vi "VERIFY DATA.vi"(11 "DATA IN":T1[](array[typedef])) -> (2 "DATA BAD?":bool, 3 "DATA OUT":T1[](array[typedef]))   [LabVIEW 2019]
uses:
  Controls/Table Data Types/Inventory Data Type.ctl
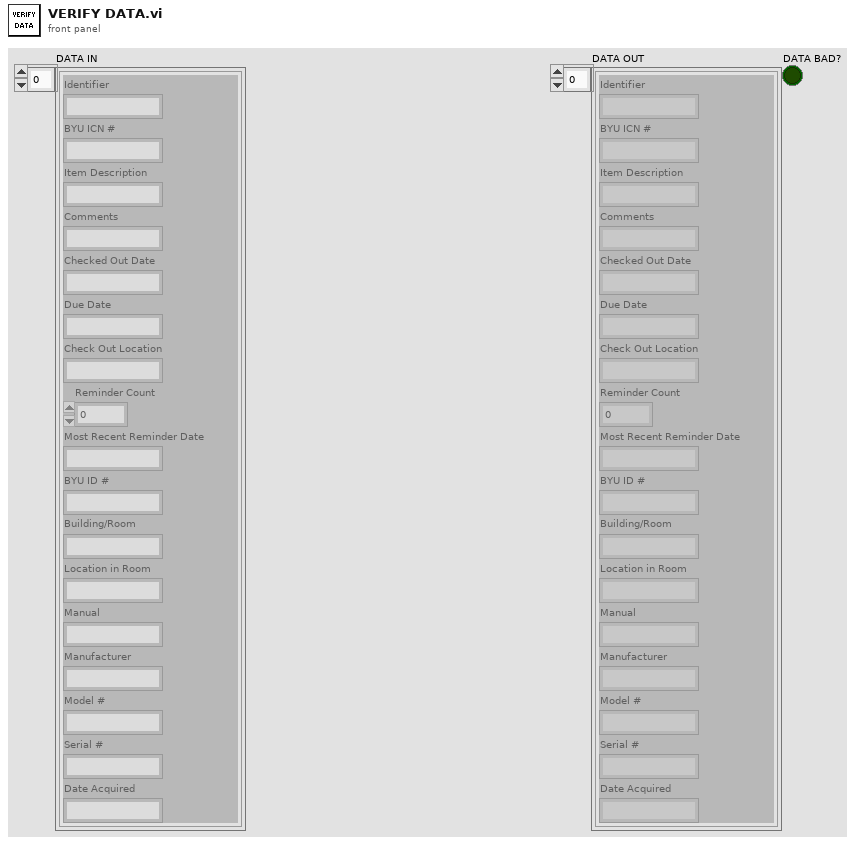
[diagram p1: front panel]
types:
  T1 = typedef "Inventory Data Type.ctl" = cluster{"Identifier":string, "BYU ICN #":string, "Item Description":string, "Comments":string, "Checked Out Date":string, "Due Date":string, "Check Out Location":string, "Reminder Count":i32, "Most Recent Reminder Date":string, "BYU ID #":string, "Building/Room":string, "Location in Room":string, "Manual":string, "Manufacturer":string, "Model #":string, "Serial #":string, "Date Acquired":string}
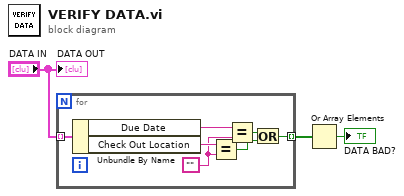
[diagram p0: block diagram]
diagram:
  n1 = for {
    tunnel: "DATA IN" -> [w10] mode=indexing
    tunnel: [w4] -> w2 mode=indexing
    w7 = ""
    n2 = Unbundle By Name(w10) -> ("Due Date"=w9:string, "Check Out Location"=w8:string)
    n3 = Equal?(x=w8, y=w7) -> (x = y?=w5:bool)
    n4 = Equal?(x=w9, y=w7) -> (x = y?=w6:bool)
    n5 = Or(x=w6, y=w5) -> (x .or. y?=w4:bool)
  }
  n6 = Or Array Elements(Boolean array=w2) -> (logical OR=→"DATA BAD?":bool)
  "DATA OUT" <- "DATA IN"
